vi "Dashboard Main.vi"() -> ()   [LabVIEW 2015]
uses:
  Camera Types.ctl
  <vilib>/Utility/miscctls.llb/LVRowAndColumnTypeDef.ctl
  <vilib>/event_ctls.llb/eventvkey.ctl
  <vilib>/Rock Robotics/WPI/Dashboard/WPI_DashboardLogging Global.vi
  <vilib>/Utility/file.llb/Write Delimited Spreadsheet (DBL).vi
  <vilib>/Rock Robotics/Network Tables/NT Write Numeric Array.vi
  <vilib>/Utility/file.llb/Read Delimited Spreadsheet (DBL).vi
  <vilib>/Rock Robotics/Network Tables/NT Read Boolean.vi
  <vilib>/Utility/config.llb/Write Key (String).vi
  <vilib>/Utility/config.llb/Write Key (I32).vi
  <vilib>/Utility/config.llb/NI_LVConfig.lvlib
  <vilib>/vision/NI_Vision_Development_Module.lvlib
panel:
  in  "Dashboard Tab":T1(tab)=enum."Camera Settings"
  out "Have ball?":bool
  out "Gyro":dbl
  in  "Camera Settings":T2={"Frame Rate"=30, "Compression"=30, "Size"=1} {"Frame Rate" scale=1.0..30.0; "Size" items=["640x480", "320x240", "160x120"]}
  out "Mode":T3(ring)=enum."Auto Disabled"
  in  "DB Camera Config":bool
  out "fps":dbl format="%#.1g"
  out "Mbps":dbl format="%#.1g"
  out "Mbps LED":bool
  in  "Auto Position":i32(slide)=1 scale=1.0..5.0
  in  "Auto Defense":T4(ring)=enum."Low Bar"
  out "TARGET":dbl
  in  "Test Slider":dbl(slide) scale=0.0..100.0 scale format="%#_3g"
  in  "On/Off":bool caption="Solenoid"
  in  "Test Name":u16(ring) items=["Select the test to run..."]
  in  "Test Tree":string(tree)
  in  "Motor":cluster{"Value":dbl, "Enable":bool} {"Value" scale=-1.0..1.0 scale format="%#_3g"}
  out "Progress":T5 {"Test Progress" scale=0.0..100.0}
  in  "Rev/Fwd":cluster{"Forward":bool, "Reverse":bool}
  in  "Test Ring":u16(ring) items=["Monochrome", "Color"]
  out "Cmd Status":string
  in  "Execute Command":bool
  in  "Command Params":string[][](table)
  in  "Command Selection":i32(listbox)
  out "NT Connection":bool
  in  "Select Auto":string(combo)
  in  "CheckList":i32(listbox)
  out "Detected Targets":T6(array[cluster]) {"Normalized Rect"."Numeric 5" format="%#_2g"; "Normalized Rect"."Numeric 3" format="%#_2g"; "Normalized Rect"."Numeric 2" format="%#_2g"; "Normalized Rect"."Numeric" format="%#_2g"}
  out "Masked":T7(plugin-control)
  out "Background":bool
  out "Qualified Particles":i32
  out "Highest Avg Score":dbl format="%#_3g"
  in  "Std Devs for Calibration":cluster{"H":dbl, "S":dbl, "V":dbl}={"H"=4.0, "S"=6.0, "V"=6.0}
  in  "Rec Mode":enum32{"Stop", "Record", "Playback"}(radio)
  in  "LED Color":T8={"Hue"={110.52399131877658, 148.6727294921875}, "Sat"={34.78571428571429, 255.0}, "Val"={91.07142857142858, 255.0}} {"Hue" scale=0.0..255.0 scale format="%_1f"}
  in  "Annotate":bool=TRUE
  in  "Annotation Limit":dbl=75.0
  in  "Aspect Ratio Fudge Factor":dbl=1.0
  in  "Min Score Threshold":i32=70
  in  "Camera Type":T9=enum."1013"
  in  "Emphasize Limit Tests":bool=TRUE
  in  "Green BCG Values":T10={"Brightness"=128.0, "Contrast"=45.0, "Gamma"=1.0} {"Brightness" min=0 max=255 step=1 format="%.2f"; "Contrast" min=1 max=89 step=1 format="%.2f"; "Gamma" min=0.1 max=10 step=0.01 format="%.2f"}
  in  "Blue BCG Values":T10={"Brightness"=128.0, "Contrast"=45.0, "Gamma"=1.0} {"Brightness" min=0 max=255 step=1 format="%.2f"; "Contrast" min=1 max=89 step=1 format="%.2f"; "Gamma" min=0.1 max=10 step=0.01 format="%.2f"}
  in  "Red BCG Values":T10={"Brightness"=128.0, "Contrast"=45.0, "Gamma"=1.0} {"Brightness" min=0 max=255 step=1 format="%.2f"; "Contrast" min=1 max=89 step=1 format="%.2f"; "Gamma" min=0.1 max=10 step=0.01 format="%.2f"}
  in  "Vision":u16(ring) items=["Camera Off", "USB Camera SW", "USB Camera HW", "IP Camera"]
  in  "Save?":bool
  out "Tree":string(tree)
  out "Original Image":T7(plugin-control)
  out "Camera Image":T7(plugin-control)
  in  "TCP":refnum<k5>
  out "Camera IP":string
  out "Image Message":string="Timeout in Camera Communications"
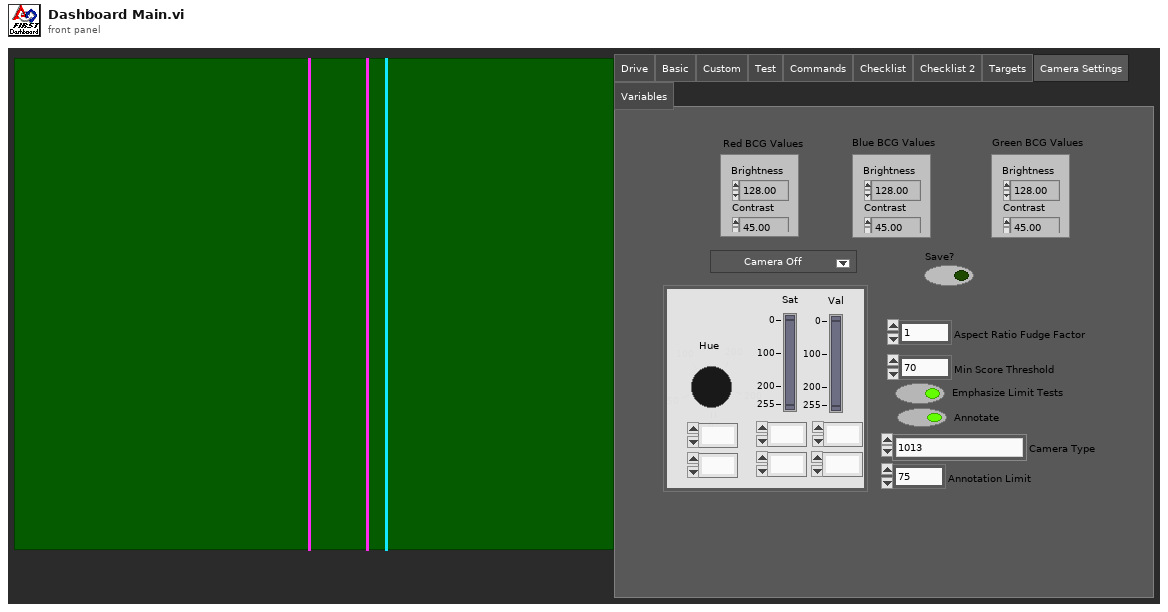
[diagram p1: front panel]
types:
  T1 = enum32{"Drive", "Basic", "Custom", "Test", "Commands", "Checklist", "Checklist 2", "Targets", "Camera Settings", "Variables"}
  T2 = cluster{"Frame Rate":i32, "Compression":i32, "Size":u16}
  T3 = enum8{"Tele-Op Disabled", "Tele-Op Enabled", "Auto Disabled", "Auto Enabled", "Test Disabled", "Test Enabled", "Disconnected", "No Code", "E-Stop"}
  T4 = enum16{"Portcullis", "Cheval de Frise", "Low Bar", "Rock Wall", "Rough Terrain", "Moat", "Ramparts", "2-ball"}
  T5 = cluster{"Test Progress":u8, "Test Progress Text":string}
  T6 = cluster{"Distance (ft)":dbl, "Center":cluster{dbl, dbl}, "Normalized Rect":cluster{"Numeric":dbl, "Numeric 2":dbl, "Numeric 3":dbl, "Numeric 5":dbl}}[]
  T7 = typedef "IMAQ Image.ctl" = refnum<image>
  T8 = cluster{"Hue":cluster{dbl, dbl}, "Sat":cluster{dbl, dbl}, "Val":cluster{dbl, dbl}}
  T9 = typedef "Camera Types.ctl" = enum16{"206", "1011", "1013", "MS HD3000 square", "MS HD3000 640x480"}
  T10 = cluster{"Brightness":sgl, "Contrast":sgl, "Gamma":sgl}
  T11 = typedef "Image Type" = u32
  T12 = cluster{"IDs":cluster{"RPC field ID":u16, "Unique ID":u16}, "String":string}
  T13 = enum32{"Drive", "Basic", "Custom", "Test", "Checklist", "Variables"}
  T14 = cluster{cluster{"Numeric":dbl, "Numeric":dbl}, cluster{"Numeric":dbl, "Numeric":dbl}, cluster{"Numeric":dbl, "Numeric":dbl}}
  T15 = cluster{"Camera Image":refnum<vi>, "Dashboard Tab":refnum<vi>, "Background":refnum<vi>, "Vision":refnum<vi>, "Rec Mode":refnum<vi>, "Test Slider":refnum<vi>, "On/Off ":refnum<vi>, "Test Ring":refnum<vi>, "Rev/Fwd":refnum<vi>, "Test Name":refnum<vi>, "Motor":refnum<vi>, "Progress":refnum<vi>, "CheckList":refnum<vi>, "Tree":refnum<vi>, "Test Tree":refnum<vi>, "Command Params":refnum<vi>, "Command Selection":refnum<vi>, "Execute Command":refnum<vi>, "Cmd Status":refnum<vi>}
  T16 = typedef "Particle Parameters" = i32
  T17 = cluster{cluster{dbl, dbl}, cluster{dbl, dbl}, cluster{dbl, dbl}}
  T18 = cluster{"Bounding box":cluster{"left":dbl, "top":dbl, "right":dbl, "bottom":dbl}, "Aspect Ratio":dbl, "Area to CH":dbl, "X Mask":dbl, "Y Mask":dbl, "Moment":dbl}[]
  T19 = cluster{"Distance (ft)":dbl, "Center":cluster{dbl, dbl}, "Normalized Rect":cluster{"Numeric":dbl, "Numeric 2":dbl, "Numeric 3":dbl, "Numeric 5":dbl}}
  T20 = cluster{"Numeric":dbl, "Numeric 2":dbl, "Numeric 3":dbl, "Numeric 5":dbl}
  T21 = typedef "NI_LVConfig.lvlib/Config Data RefNum.ctl" = refnum<k1>
  T22 = cluster{"Error Strings":string, "Disable Counts":cluster{u16, u16}, "Rail Faults":cluster{u16, u16, u16}, "Robot IP":string, "DB Mode":u8, "Event Info":cluster{"Name":string, "Type":u8, "Number":u16, "Replay":u8}, "Camera Addr":string}
  T23 = cluster{"Storage":cluster{"Disk Free":u64, "RAM Block":u32, "RAM free":u32}, "CPU Utilization":cluster{"CPU % ISR":sgl, "CPU % Time Crit":sgl, "CPU % Timed Str":sgl, "CPU % High":sgl, "CPU % Above":sgl, "CPU % Normal":sgl, "CPU % Low":sgl}, "CAN":cluster{"% Bus Utilization":sgl, "Bus Off Cnt":u32, "TX_FIFO Full Cnt":u32, "Receive Error Cnt":u8, "Transmit Error Cnt":u8}, "HID":cluster{"HID Outputs":u32, "Rumble Low":u16, "Rumble High":u16}[]}
  T24 = cluster{"Status bits":cluster{"Test Mode":bool, "Autonomous":bool, "Enabled":bool, "Code Start":bool, "Brownout":bool, "Reserved 2":bool, "Reserved 3":bool, "E-Stop":bool}, "Code Trace":cluster{"Disabled":bool, "TeleOp":bool, "Auto":bool, "Test":bool}, "Controller Type":enum16{"unknown", "cRIO", "roboRio"}, "Code?":enum16{"unknown", "noCode", "code"}, "Battery V":dbl}
  T25 = cluster{"Control Bits":cluster{"TestMode":bool, "Autonomous":bool, "Enabled":bool, "FMS Present":bool, bool, bool, bool, "E-Stop":bool}, "Team Station ":u8, "Countdown":sgl, "Joystick Values":cluster{"Axes":dbl[], "Buttons":bool[], "POVs":i16[]}[]}
  T26 = cluster{"Operation":enum16{"Update", "Clear"}, "Color Box":u32}[]
  T27 = typedef "eventvkey.ctl" = enum16{"ASCII", "Enter", "Return", "Shift", "Ctrl", "Alt", "Cmd", "Opt", "Caps", "NumLock", "Clear", "Break", "Up", "Down", "Left", "Right", "Insert", "Delete", "Home", "End", "PageUp", "PageDown", "Escape", "Help", "Pause", "ScrollLock", "F1", "F2", "F3", "F4", "F5", "F6", "F7", "F8", "F9", "F10", "F11", "F12", "F13", "F14", "F15", "F16", "F17", "F18", "F19", "F20", "F21", "F22", "F23", "F24", "Play", "VolumeUp", "VolumeDown", "Mute", "Two Byte Char"}
  T28 = cluster{"Image Size":bool, "Image Type":bool, "Pixel Value":bool, "ROI Information":bool, "Zoom Factor":bool}
  T29 = enum8{"Enabled", "Disabled", "Disabled and Grayed Out"}
  T30 = cluster{"Operation":enum16{"Update", "Clear"}, "Color Box":u32}
  T31 = typedef "LVRowAndColumnTypeDef.ctl" = cluster{"Row":i32, "Column":i32}
  T32 = cluster{"Shift":bool, "Ctrl":bool, "Alt":bool, "Cmd":bool, "Opt":bool}
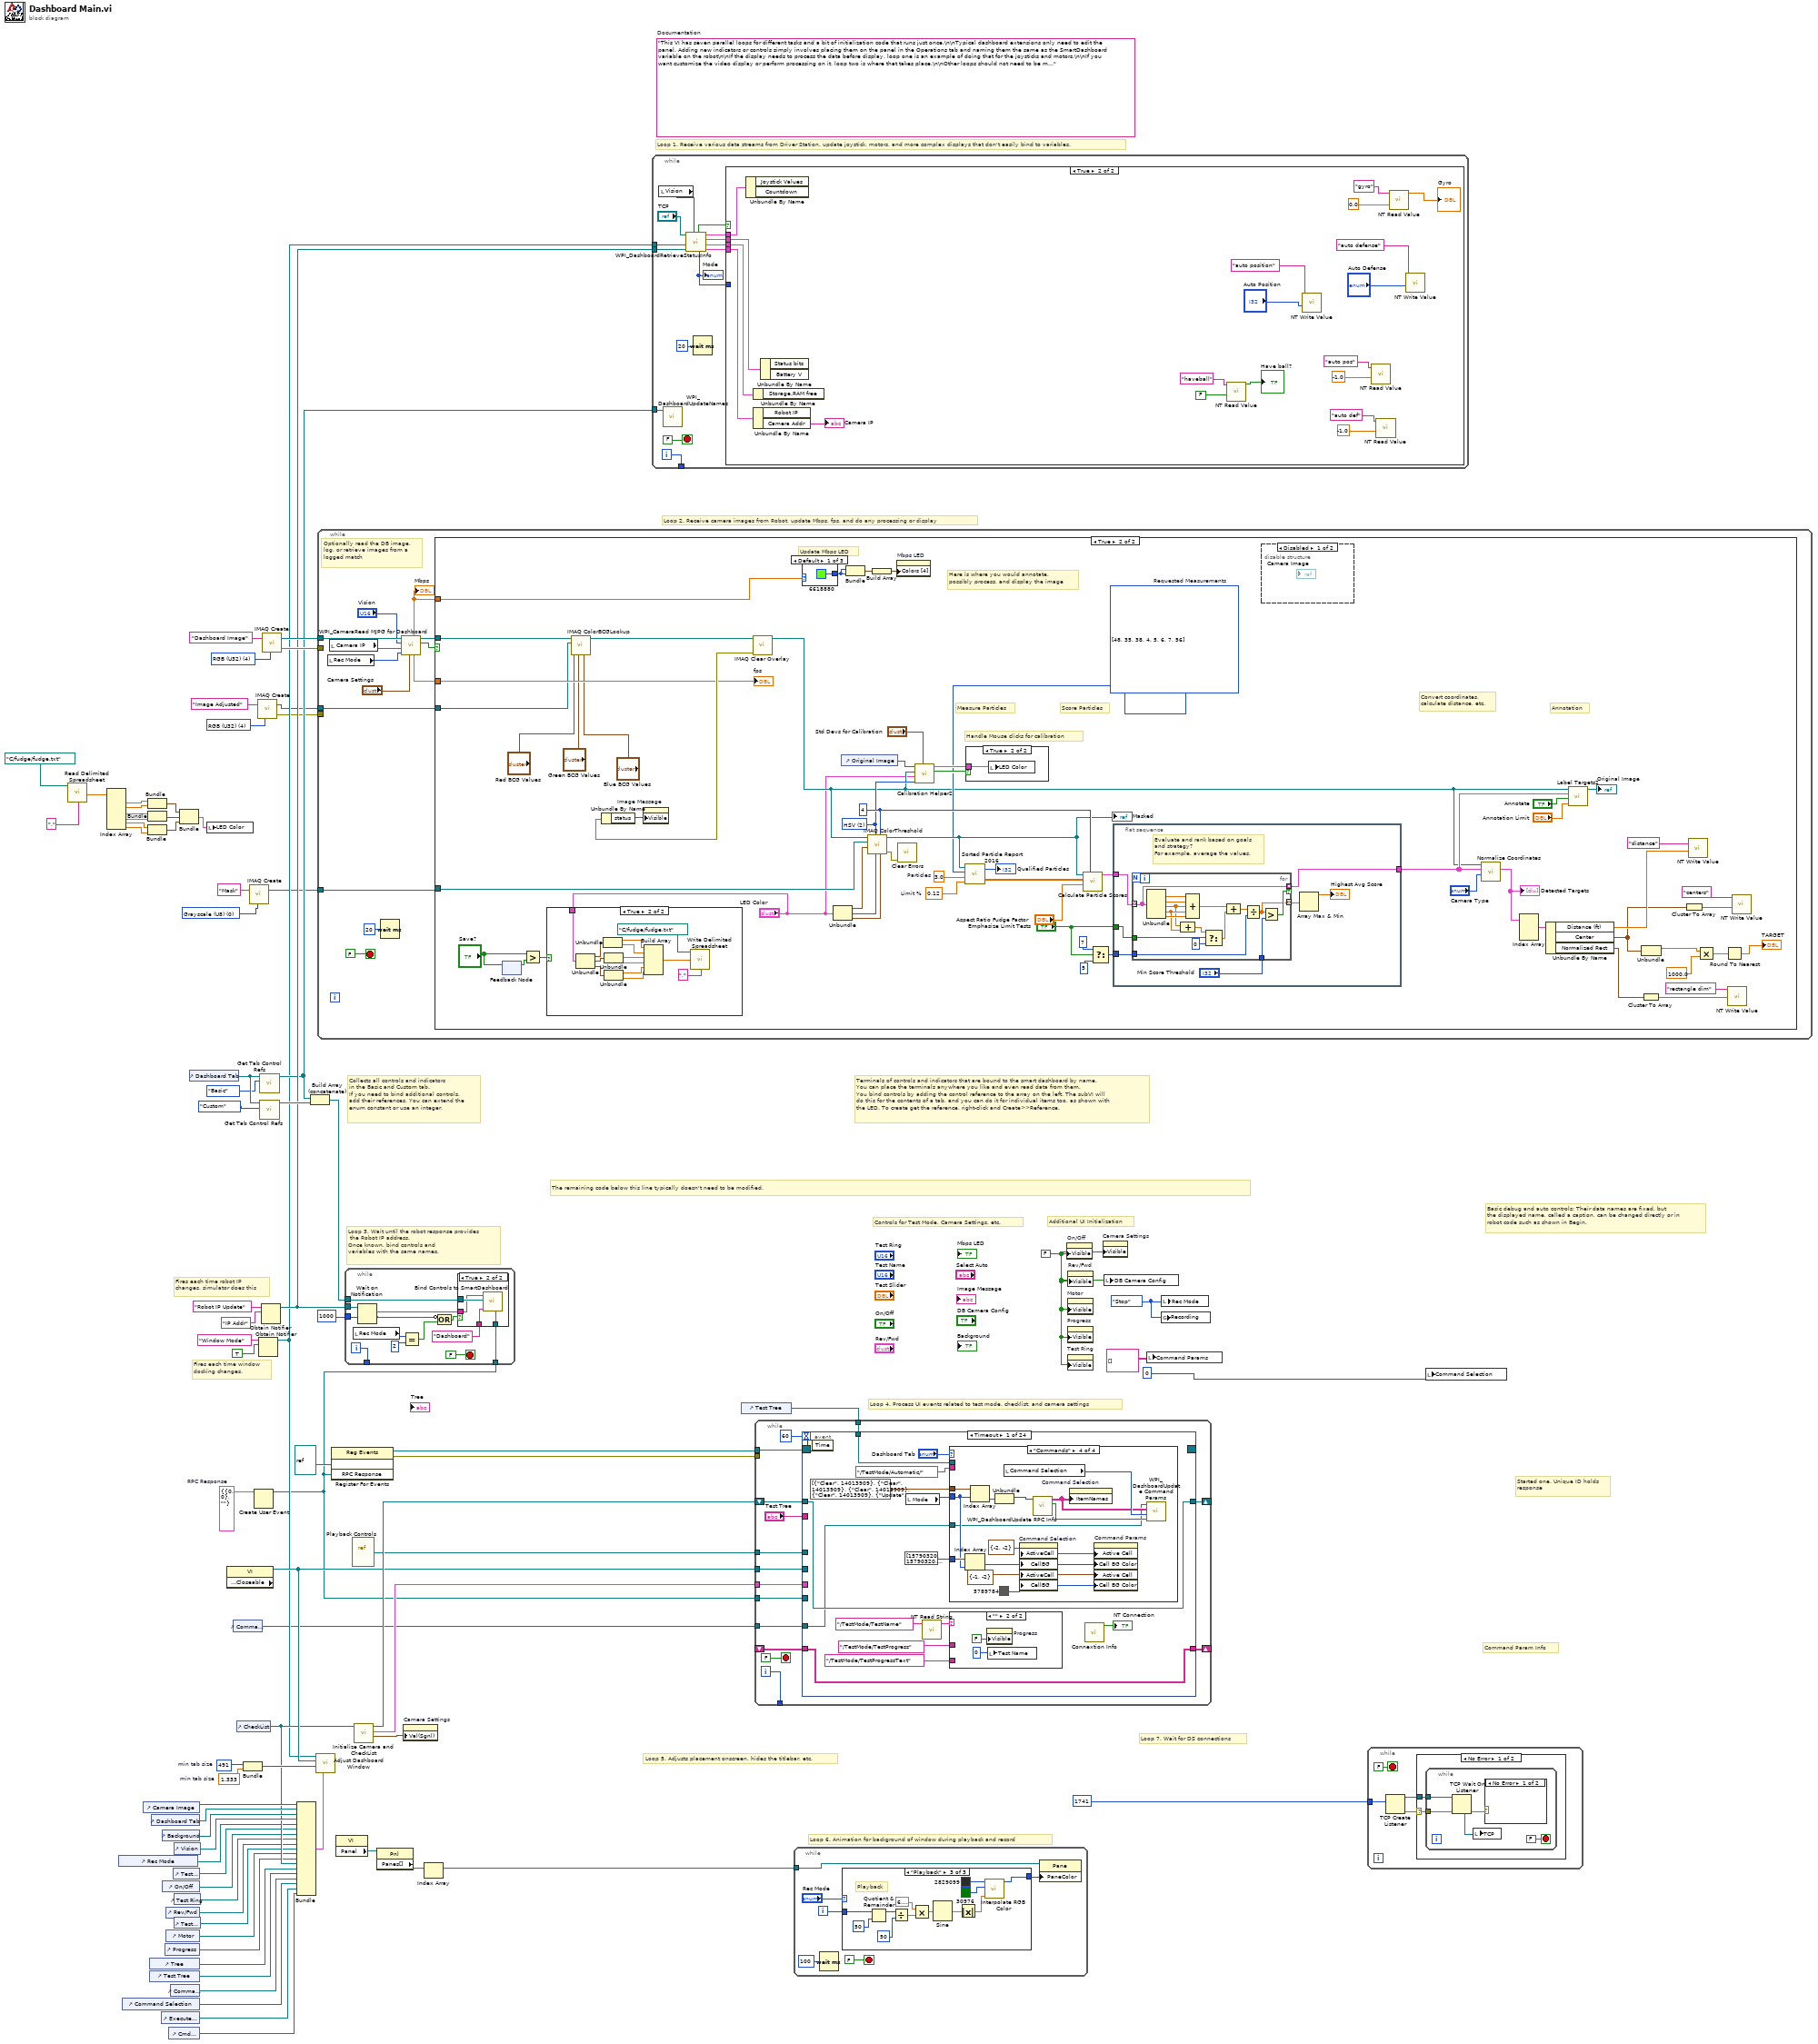
[diagram p0: block diagram]
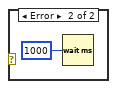
[diagram p2: hidden frame]
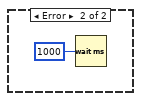
[diagram p3: hidden frame]
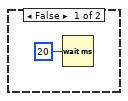
[diagram p4: hidden frame]
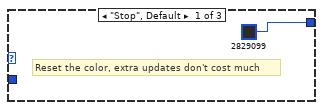
[diagram p5: hidden frame]
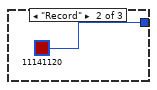
[diagram p6: hidden frame]
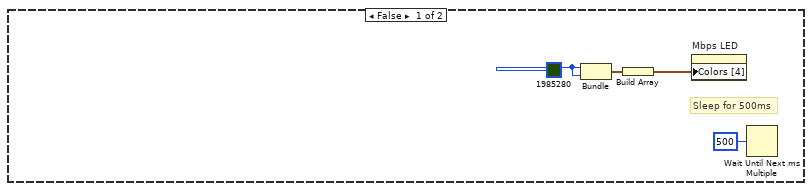
[diagram p8: hidden frame]
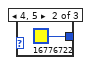
[diagram p12: hidden frame]
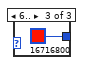
[diagram p13: hidden frame]
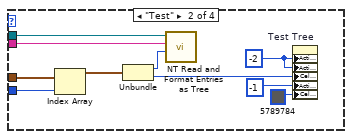
[diagram p15: hidden frame]
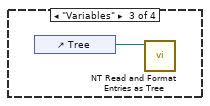
[diagram p16: hidden frame]
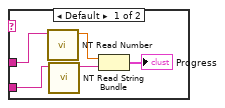
[diagram p17: hidden frame]
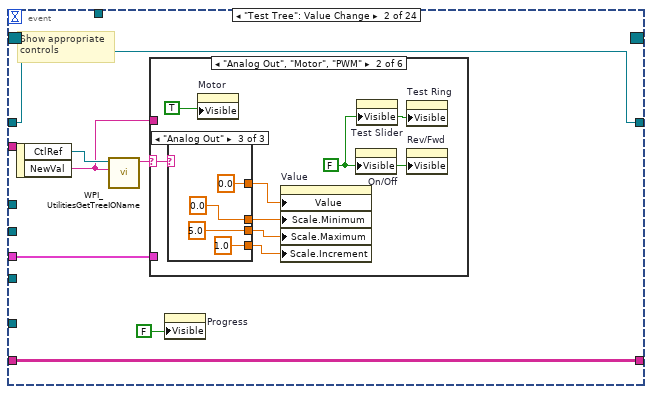
[diagram p18: hidden frame]
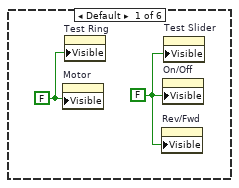
[diagram p19: hidden frame]
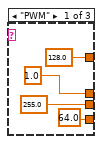
[diagram p20: hidden frame]
diagram:
  w17 = T11 4 items=["Grayscale (U8)", "Grayscale (I16)", "Grayscale (SGL)", "Complex (CSG)", "RGB (U32)", "HSL (U32)", "RGB (U64)"] ("Image Type")
  w19 = T11 0 items=["Grayscale (U8)", "Grayscale (I16)", "Grayscale (SGL)", "Complex (CSG)", "RGB (U32)", "HSL (U32)", "RGB (U64)", "Grayscale (U16)"] ("Image Type")
  w27 = T12 {"IDs"={"RPC field ID"=0, "Unique ID"=0}, "String"=""}  # RPC Response
  w52 = 491  # min tab size
  w51 = 1.333  # min tab size
  w60 = enum32{"Stop", "Record", "Playback"}."Stop" ("Rec Mode")
  w34 = FALSE ("Visible")
  (unwired) "This VI has seven parallel loops for different tasks and a bit of initialization code that runs just once.\n\nTypical dashboard extensions only need to edit the panel. Adding new indicators or controls simply involves placing them on the panel in the Operations tab and naming them the same as the SmartDashboard variable on the robot\n\nIf the display needs to process the data before display, loop one is an example of doing that for the joysticks and motors.\n\nIf you want customize the video display or perform processing on it, loop two is where that takes place.\n\nOther loops should not need to be modified. They are pretty standard, and document the task they perform."  # Documentation
  w80 = T11 4 items=["Grayscale (U8)", "Grayscale (I16)", "Grayscale (SGL)", "Complex (CSG)", "RGB (U32)", "HSL (U32)", "RGB (U64)"] ("Image Type")
  # "Command Param Info"
  # "Started one, Unique ID holds\nresponse"
  # "Loop 7. Wait for DS connections"
  # "Basic debug and auto controls: Their data names are fixed, but\nthe displayed name, called a caption, can be changed directly or in\nrobot code such as shown in Begin."
  # "Controls for Test Mode, Camera Settings, etc."
  # "Additional UI Initialization"
  # "Loop 6. Animation for background of window during playback and record"
  # "Fires each time robot IP\nchanges, simulator does this"
  # "Fires each time window\ndocking changes."
  # "Collects all controls and indicators\nin the Basic and Custom tab.\nIf you need to bind additional controls,\nadd their references. You can extend the\nenum constant or use an integer."
  # "The remaining code below this line typically doesn't need to be modified."
  # "Loop 4. Process UI events related to test mode, checklist, and camera settings"
  # "Terminals of controls and indicators that are bound to the smart dashboard by name.\nYou can place the terminals anywhere you like and even read data from them.\nYou bind controls by adding the control reference to the array on the left. The subVI will\ndo this for the contents of a tab, and you can do it for individual items too, as shown with\nthe LED. To create get the reference, right-click and Create>>Reference."
  # "Loop 3. Wait until the robot response provides\n the Robot IP address.\nOnce known, bind controls and\nvariables with the same names."
  # "Loop 5. Adjusts placement onscreen, hides the titlebar, etc."
  # "Loop 1. Receive various data streams from Driver Station, update joystick, motors, and more complex displays that don't easily bind to variables."
  # "Loop 2. Receive camera images from Robot, update Mbps, fps, and do any processing or display"
  n1 = call-poly <vilib>:"Read Delimited Spreadsheet.vi"("file path (dialog if empty)"=path "C:/fudge/fudge.txt", "delimiter (\\t)"="," ("delimiter (\\t)")) -> ("first row"=w11:dbl[])  [unwired: 8 in, 5 out]
  n2 = Index Array(array=w11) -> (element #1=w10:dbl, element #2=w9:dbl, element #3=w8:dbl, element #4=w7:dbl, element #5=w6:dbl, element #6=w5:dbl)  [unwired: 6 in]
  n3 = control-ref of="Rec Mode"() -> (w40:refnum<vi>)
  n4 = control-ref of="Command Selection"() -> (w26:refnum<vi>)
  n5 = control-ref of="Camera Image"() -> (w55:refnum<vi>)
  n6 = Bundle("Numeric"=w10, "Numeric"=w9) -> (w4:cluster{"Numeric":dbl, "Numeric":dbl})  [unwired: 1 in]
  n7 = Bundle("Numeric"=w8, "Numeric"=w7) -> (w3:cluster{"Numeric":dbl, "Numeric":dbl})  [unwired: 1 in]
  n8 = Bundle("Numeric"=w6, "Numeric"=w5) -> (w2:cluster{"Numeric":dbl, "Numeric":dbl})  [unwired: 1 in]
  n9 = control-ref of="Tree"() -> (w44:refnum<vi>)
  n10 = control-ref of="Test Tree"() -> (w43:refnum<vi>)
  n11 = control-ref of="Dashboard Tab"() -> (w54:refnum<vi>)
  n12 = control-ref of="Execute Command"() -> (w28:refnum<vi>)
  n13 = control-ref of="Background"() -> (w49:refnum<vi>)
  n14 = control-ref of="On/Off"() -> (w38:refnum<vi>)
  n15 = control-ref of="Progress"() -> (w35:refnum<vi>)
  n16 = control-ref of="Rev/Fwd"() -> (w36:refnum<vi>)
  n17 = control-ref of="Motor"() -> (w41:refnum<vi>)
  n18 = control-ref of="Cmd Status"() -> (w22:refnum<vi>)
  n19 = control-ref of="Command Params"() -> (w29:refnum<vi>)
  n20 = control-ref of="Test Slider"() -> (w39:refnum<vi>)
  n21 = control-ref of="Vision"() -> (w53:refnum<vi>)
  n22 = control-ref of="Test Ring"() -> (w37:refnum<vi>)
  n23 = control-ref of="Test Name"() -> (w42:refnum<vi>)
  n24 = Bundle(w4, w3, w2) -> (w1:T14)  [unwired: 1 in]
  n25 = control-ref of="Dashboard Tab"() -> (w58:refnum<vi>)
  n26 = local write "LED Color"(w1) -> ()
  n27 = property class="VI" props=["Front Panel.Closeable"]() -> (reference out=w59:refnum<vi>)  [unwired: 2 in, 2 out]
  n28 = control-ref of="Command Params"() -> (w21:refnum<vi>)
  n29 = control-ref of="CheckList"() -> (w45:refnum<vi>)
  n30 = Bundle("min tab size"=w52, "min tab size"=w51) -> (w50:cluster{"min tab size":i32, "min tab size":dbl})  [unwired: 1 in]
  n31 = call "IMAQ Create"("Image Name"="Mask", "Image Type"=w19) -> ("New Image"=w18:T7)  [unwired: 2 in, 2 out]
  n32 = Create User Event(user event datatype=w27) -> (user event=w23:refnum<user-event>)  [unwired: 1 in, 1 out]
  n33 = call "IMAQ Create"("Image Name"="Image Adjusted", "Image Type"=w17) -> ("New Image"=w15:T7, "error out"=w14:errorcluster)  [unwired: 2 in, 1 out]
  n34 = Obtain Notifier(name (unnamed)="Window Mode", notification data type=TRUE) -> (notifier out=w31:refnum<notifier>)  [unwired: 2 in, 2 out]
  n35 = call <vilib>:"Get Tab Control Refs.vi"("Page Index"=T13."Basic" ("Dashboard Tab"), "TabControl in"=w58) -> ("ControlsOnPage"=w32:refnum<vi>[])  [unwired: 9 in]
  n36 = call <vilib>:"Get Tab Control Refs.vi"("Page Index"=T13."Custom" ("Dashboard Tab"), "TabControl in"=w58) -> ("ControlsOnPage"=w57:refnum<vi>[])  [unwired: 9 in]
  n37 = Obtain Notifier(name (unnamed)="Robot IP Update", notification data type="IP Addr" ("name (unnamed)")) -> (notifier out=w33:refnum<notifier>)  [unwired: 2 in, 2 out]
  n38 = call "IMAQ Create"("Image Name"="Dashboard Image", "Image Type"=w80) -> ("New Image"=w78:T7, "error out"=w77:errorcluster)  [unwired: 2 in, 1 out]
  n39 = Bundle("Camera Image"=w55, "Dashboard Tab"=w54, "Background"=w49, "Vision"=w53, "Rec Mode"=w40, "Test Slider"=w39, "On/Off"=w38, "Test Ring"=w37, "Rev/Fwd"=w36, "Test Name"=w42, "Motor"=w41, "Progress"=w35, "CheckList"=w45, "Tree"=w44, "Test Tree"=w43, "Command Params"=w29, "Command Selection"=w26, "Execute Command"=w28, "Cmd Status"=w22) -> (w46:T15)  [unwired: 1 in]
  n40 = Build Array (concatenate)(w32, w57) -> (w56:refnum<vi>[])
  n41 = call "Adjust Dashboard Window.vi"("Sizing Refnums"=w46, "Size Constraints"=w50, "VI"=w59, "WIn Mode"=w31) -> ()  [unwired: 8 in]
  n42 = while {
    tunnel: w78 -> [w93]
    tunnel: w77 -> [_]
    tunnel: w18 -> [w83]
    tunnel: w15 -> [w82]
    tunnel: w14 -> [_]
    stop <- FALSE stop-if-true
    # "Optionally read the DB image,\nlog, or retrieve images from a\nlogged match"
    n43 = local read "Rec Mode"() -> (w88:enum32{"Stop", "Record", "Playback"})
    n44 = local read "Camera IP"() -> (w86:string)
    n45 = Wait (ms)(milliseconds to wait=u32 20) -> ()  [unwired: 1 out]
    n46 = call <vilib>:"WPI_CameraRead MJPG for Dashboard.vi"("Camera Settings"="Camera Settings", "Rec Mode"=w88, "Camera IP"=w86, "Camera Mode"="Vision", "Refnum in"=w93) -> ("Active"=w91:bool, "Refnum out"=w92:T7, "FPS"=w90:dbl, "Bandwidth (Mbps)"=w85:dbl)  [unwired: 3 in]
    "Mbps" <- w85
    n47 = case shown="True" w91 {
      tunnel: w92 -> [_ w121]
      tunnel: w85 -> [_ w152]
      tunnel: w90 -> [_ w151]
      tunnel: w83 -> [_ w125]
      tunnel: w82 -> [_ w119]
      frame False {
        w94 = u32 1985280 ("Color Box")
        # "Sleep for 500ms"
        n48 = Bundle("Color Box"=w94, "Color Box"=w94) -> (w96:cluster{"Color Box":u32, "Color Box":u32})  [unwired: 1 out]
        n49 = Build Array(w96) -> (w95:cluster{"Color Box":u32, "Color Box":u32}[])
        n50 = property on="Mbps LED" class="Bool (strict)"("Colors [4]"=w95) -> ()  [unwired: 2 in, 2 out]
        n51 = Wait Until Next ms Multiple(millisecond multiple=u32 500) -> ()  [unwired: 1 out]
      }
      frame True {
        w124 = T16[] [48, 35, 38, 4, 5, 6, 7, 56] items=["Center of Mass X", "Center of Mass Y", "First Pixel X", "First Pixel Y", "Bounding Rect Left", "Bounding Rect Top", "Bounding Rect Right", "Bounding Rect Bottom", "Max Feret Diameter Start X", "Max Feret Diameter Start Y", "Max Feret Diameter End X", "Max Feret Diameter End Y", "Max Horiz. Segment Length Left", "Max Horiz. Segment Length Right", "Max Horiz. Segment Length Row", "-", "Bounding Rect Width", "Bounding Rect Height", "Bounding Rect Diagonal", "Perimeter", "Convex Hull Perimeter", "Holes' Perimeter", "Max Feret Diameter", "Equivalent Ellipse Major Axis", "Equivalent Ellipse Minor Axis", "Equivalent Ellipse Minor Axis (Feret)", "Equivalent Rect Long Side", "Equivalent Rect Short Side", "Equivalent Rect Diagonal", "Equivalent Rect Short Side (Feret)", "Average Horiz. Segment Length", "Average Vert. Segment Length", "Hydraulic Radius", "Waddel Disk Diameter", "-", "Area", "Holes' Area", "Particle & Holes' Area", "Convex Hull Area", "Image Area", "-", "Number of Holes", "Number of Horiz. Segments", "Number of Vert. Segments", "-", "Orientation", "Max Feret Diameter Orientation", "-", "% Area/Image Area", "% Area/(Particle & Holes' Area)", "Ratio of Equivalent Ellipse Axes", "Ratio of Equivalent Rect Sides", "-", "Elongation Factor", "Compactness Factor", "Heywood Circularity Factor", "Type Factor", "-", "Sum X", "Sum Y", "Sum XX", "Sum XY", "Sum YY", "Sum XXX", "Sum XXY", "Sum XYY", "Sum YYY", "-", "Moment of Inertia XX", "Moment of Inertia XY", "Moment of Inertia YY", "Moment of Inertia XXX", "Moment of Inertia XXY", "Moment of Inertia XYY", "Moment of Inertia YYY", "Norm. Moment of Inertia XX", "Norm. Moment of Inertia XY", "Norm. Moment of Inertia YY", "Norm. Moment of Inertia XXX", "Norm. Moment of Inertia XXY", "Norm. Moment of Inertia XYY", "Norm. Moment of Inertia YYY", "Hu Moment 1", "Hu Moment 2", "Hu Moment 3", "Hu Moment 4", "Hu Moment 5", "Hu Moment 6", "Hu Moment 7"]  # Requested Measurements
        w142 = 4 ("Replace Value")
        w144 = 0.12  # Limit %
        w147 = 3.0  # Particles
        w128 = u16 2 items=["RGB", "HSL", "HSV", "HSI"] ("Color Mode")
        # "Handle Mouse clicks for calibration"
        # "Measure Particles"
        # "Convert coordinates,\ncalculate distance, etc."
        # "Annotation"
        # "Score Particles"
        # "Here is where you would annotate,\npossibly process, and display the image"
        # "Update Mbps LED"
        n52 = feedback-in #1("Save?") -> ()
        n53 = feedback #1() -> (w100:bool)  [unwired: 1 in]
        n54 = Greater?(x="Save?", y=w100) -> (0:w101:bool)
        n55 = case shown="True" w101 {
          tunnel: "LED Color" -> [_ w162]
          frame False {
          }
          frame True {
            n56 = Unbundle(w162) -> ("Hue"=w164:cluster{dbl, dbl}, "Sat"=w163:cluster{dbl, dbl}, "Val"=w161:cluster{dbl, dbl})
            n57 = Unbundle(w164) -> (w170:dbl, w169:dbl)
            n58 = Unbundle(w163) -> (w168:dbl, w167:dbl)
            n59 = Unbundle(w161) -> (w166:dbl, w165:dbl)
            n60 = Build Array(w170, w169, w168, w167, w166, w165) -> (w159:dbl[])
            n61 = call-poly <vilib>:"Write Delimited Spreadsheet.vi"("file path (dialog if empty)"=path "C:/fudge/fudge.txt", "1D data"=w159, "delimiter (\\t)"="," ("delimiter (\\t)")) -> ()  [unwired: 11 in, 2 out]
          }
        }
        n62 = call "IMAQ ColorBCGLookup"("Blue BCG Values"="Blue BCG Values", "Green BCG Values"="Green BCG Values", "Red BCG Values"="Red BCG Values", "Image Dst"=w119, "Image Src"=w121) -> ("Image Dst Out"=w120:T7)  [unwired: 5 in, 1 out]
        n63 = call "IMAQ Clear Overlay"("Image"=w120) -> ("error out"=w156:errorcluster, "Image Out"=w122:T7)  [unwired: 2 in, 7 out]
        n64 = Unbundle By Name(w156) -> ("status"=w157:bool)
        n65 = property on="Image Message" class="Str"("Visible"=w157) -> ()  [unwired: 2 in, 2 out]
        n66 = case shown="Default" w152 {
          tunnel: [u32 6618880 ("Color Box") u32 16776722 ("Color Box") u32 16716800 ("Color Box")] -> w153
          frame Default {
          }
          frame 4, 5 {
          }
          frame 6.. {
          }
        }
        n67 = Unbundle("LED Color") -> ("Hue"=w150:cluster{dbl, dbl}, "Sat"=w149:cluster{dbl, dbl}, "Val"=w148:cluster{dbl, dbl})
        n68 = control-ref of="Original Image"() -> (w131:refnum<vi>)
        n69 = Bundle("Color Box"=w153, "Color Box"=w153) -> (w155:cluster{"Color Box":u32, "Color Box":u32})  [unwired: 1 out]
        n70 = call "IMAQ ColorThreshold"("Blue or Luma or Val or Inten Range"=w148, "Replace Value"=w142, "Green or Sat Range"=w149, "Color Mode"=w128, "Red or Hue Range"=w150, "Image Dst"=w125, "Image Src"=w122) -> ("error out"=w135:errorcluster, "Image Dst Out"=w136:T7)  [unwired: 3 in]
        "Masked" <- w136
        n71 = Build Array(w155) -> (w154:cluster{"Color Box":u32, "Color Box":u32}[])
        n72 = property on="Mbps LED" class="Bool (strict)"("Colors [4]"=w154) -> ()  [unwired: 2 in, 2 out]
        n73 = call <vilib>:"Clear Errors.vi"("error in (no error)"=w135) -> ()  [unwired: 5 in, 2 out]
        n74 = call "Calibration Helper2.vi"("Std Devs"="Std Devs for Calibration", "Color Mode"=w128, "Color Components"="LED Color", "Image"=w122, "Image Ctl Refnum"=w131) -> ("Changed"=w130:bool, "output color"=w129:T17)  [unwired: 5 in]
        n75 = call "Sorted Particle Report 2016.vi"("Min Area Size %"=w144, "Particle Count Limit"=w147, "Pixel Measurements"=w124, "Image in"=w136) -> ("Sorted Data"=w145:dbl[][], "Particles"=→"Qualified Particles":i32)
        n76 = case shown="True" w130 {
          tunnel: w129 -> [_ w171]
          frame False {
          }
          frame True {
            n77 = local write "LED Color"(w171) -> ()
          }
        }
        n78 = call "Calculate Particle Scores.vi"("Pixel Value"=w142, "Aspect Fudge Factor"="Aspect Ratio Fudge Factor", "Sorted Data"=w145, "Image in"=w136) -> ("Scores"=w139:T18)  [unwired: 7 in]
        n79 = Select(t=7, s="Emphasize Limit Tests", f=5) -> (s? t:f=w132:i32)
        n80 = flat-sequence {
          tunnel: w139 -> [w177]
          tunnel: [w178] -> w137
          tunnel: w132 -> [w174]
          tunnel: "Emphasize Limit Tests" -> [w172]
          frame #0 {
            # "Evaluate and rank based on goals\nand strategy?\nFor example, average the values."
            n81 = for {
              tunnel: w177 -> [w192] mode=indexing
              tunnel: [w192] -> w178 mode=indexing if=w191
              tunnel: [w190] -> w176 mode=indexing
              tunnel: w174 -> [w189]
              tunnel: "Min Score Threshold" -> [w188]
              tunnel: w172 -> [w181]
              n82 = Unbundle(w192) -> ("Aspect Ratio"=w194:dbl, "Area to CH"=w193:dbl, "X Mask"=w183:dbl, "Y Mask"=w184:dbl, "Moment"=w185:dbl)  [unwired: 1 out]
              n83 = Compound Arithmetic op=ADD(w183, w184) -> (w182:dbl)
              n84 = Compound Arithmetic op=ADD(w194, w193, w183, w184, w185) -> (w187:dbl)
              n85 = Select(t=w182, s=w181, f=0) -> (s? t:f=w180:dbl)
              n86 = Compound Arithmetic op=ADD(w187, w180) -> (w186:dbl)
              n87 = Divide(x=w186, y=w189) -> (x/y=w190:dbl)
              n88 = Greater?(x=w190, y=w188) -> (0:w191:bool)
            }
            n89 = Array Max & Min(array=w176) -> (max value=→"Highest Avg Score":dbl)  [unwired: 3 out]
          }
        }
        n90 = disable-structure shown="Disabled" {
          frame Disabled {
          }
          frame Enabled {
          }
        }
        n91 = call "Normalize Coordinates.vi"("Camera Type"="Camera Type", "Targets"=w137, "Image in"=w122) -> ("Found Targets"=w115:T6)  [unwired: 7 in, 1 out]
        "Detected Targets" <- w115
        n92 = Index Array(array=w115) -> (element #1=w114:T19)  [unwired: 3 in, 2 out]
        n93 = Unbundle By Name(w114) -> ("Distance (ft)"=w112:dbl, "Center"=w106:cluster{dbl, dbl}, "Normalized Rect"=w108:T20)
        n94 = call "Label Targets2.vi"("Score Threshold"="Annotation Limit", "Annotate"="Annotate", "Targets"=w137, "Image in"=w122) -> ("Image out"=→"Original Image":T7)  [unwired: 7 in]
        n95 = Cluster To Array(cluster=w108) -> (array=w107:dbl[])
        n96 = Unbundle(w106) -> (w102:dbl)  [unwired: 1 out]
        n97 = Cluster To Array(cluster=w106) -> (array=w110:dbl[])
        n98 = call-poly <vilib>:"NT Write Value.vi"("Numeric"=w112, "Name"="distance") -> ()  [unwired: 9 in, 1 out]
        n99 = Multiply(x=w102, y=1000.0) -> (x*y=w104:dbl)
        n100 = Round To Nearest(number=w104) -> (nearest integer value=→"TARGET":dbl)
        n101 = call-poly <vilib>:"NT Write Value.vi"("Numeric Array"=w107, "Name"="rectangle dim") -> ()  [unwired: 9 in, 1 out]
        n102 = call-poly <vilib>:"NT Write Value.vi"("Numeric Array"=w110, "Name"="centers") -> ()  [unwired: 9 in, 1 out]
        "fps" <- w151
      }
    }
  }
  n103 = register-events(refnum<vi> refnum, w23) -> (reference out=w64:refnum<event-registration>, error out=w63:errorcluster)  [unwired: 2 in]
  n104 = property class="VI"() -> ("Panel"=w67:refnum<vi>)  [unwired: 2 in, 2 out]
  n105 = while {
    tunnel: w56 -> [w210]
    tunnel: w33 -> [w208]
    tunnel: [w206] -> _
    tunnel: u32 1000 ("milliseconds to wait") -> [w205]
    tunnel: w23 -> [w198]
    i -> [w206]
    stop <- FALSE stop-if-true
    n106 = local read "Rec Mode"() -> (w201:enum32{"Stop", "Record", "Playback"})
    n107 = Wait on Notification(notifier=w208, timeout in ms (-1)=w205) -> (notification=w207:string, timed out?=w203:bool)  [unwired: 2 in, 2 out]
    n108 = Equal?(x=w201, y=u16 2 ("Rec Mode")) -> (x = y?=w202:bool)
    n109 = Compound Arithmetic op=OR(invert w203, w202) -> (w204:bool)
    n110 = case shown="True" w204 {
      tunnel: w210 -> [_ w214]
      tunnel: w207 -> [_ w213]
      tunnel: "Dashboard" -> [_ w212]
      tunnel: w198 -> [_ w211]
      frame False {
      }
      frame True {
        n111 = call <vilib>:"Bind Controls to SmartDashboard.vi"("RPC ref"=w211, "Client Name"=w212, "Bound Control Refs"=w214, "Server IP Address"=w213) -> ()  [unwired: 8 in]
      }
    }
  }
  n112 = vi-ref "Playback Controls.vi"() -> (w65:refnum<vi>)
  n113 = call "Initialize Camera and CheckList.vi"("ListBox in"=w45) -> ("Cluster"=w71:cluster{"value":i32, "value":i32, "index":i32}, "Array"=w72:cluster{string[]}[], "File Refnum"=w70:T21)  [unwired: 8 in]
  n114 = property class="Pnl"(reference=w67) -> ("Panes[]"=w68:refnum<vi>[])  [unwired: 1 in, 2 out]
  n115 = property on="Camera Settings" class="Clust (strict)"("Val(Sgnl)"=w71) -> ()  [unwired: 2 in, 2 out]
  n116 = Index Array(array=w68) -> (element=w66:refnum<vi>)  [unwired: 1 in]
  n117 = while {
    tunnel: [w227] -> _
    tunnel: w33 -> [w221]
    tunnel: w32 -> [w220]
    tunnel: w31 -> [w216]
    i -> [w227]
    stop <- FALSE stop-if-true
    n118 = local read "Vision"() -> (w218:u16)
    n119 = call <vilib>:"WPI_DashboardUpdateNames.vi"("Controls on Tab"=w220) -> ()  [unwired: 11 in]
    n120 = call <vilib>:"WPI_DashboardRetrieveStatusInfo.vi"("Vision"=w218, "Binding Refnum"=w221, "Window Mode Notifier"=w216, "TCP Cnx"="TCP") -> ("Power and Errors"=w222:T22, "Robot Metrics"=w225:T23, "Status Info"=w226:T24, "Control Info"=w223:T25, "Robot Mode"=w219:T3, "Process?"=w224:bool)  [unwired: 2 in]
    "Mode" <- w219
    n121 = Wait (ms)(milliseconds to wait=u32 20) -> ()  [unwired: 1 out]
    n122 = case shown="True" w224 {
      tunnel: w226 -> [_ w248]
      tunnel: w225 -> [_ w247]
      tunnel: w223 -> [_ w246]
      tunnel: w222 -> [_ w245]
      tunnel: w219 -> [_ _]
      frame False {
        n123 = Wait (ms)(milliseconds to wait=u32 20) -> ()  [unwired: 1 out]
      }
      frame True {
        n124 = Unbundle By Name(w246) -> ()  [unwired: 2 out]
        n125 = Unbundle By Name(w247) -> ()  [unwired: 1 out]
        n126 = Unbundle By Name(w245) -> ("Camera Addr"=→"Camera IP":string)  [unwired: 1 out]
        n127 = Unbundle By Name(w248) -> ()  [unwired: 2 out]
        n128 = call-poly <vilib>:"NT Read Value.vi"("Default Value"=FALSE, "Name"="haveball") -> ("Boolean"=→"Have ball?":bool)  [unwired: 8 in, 1 out]
        n129 = call-poly <vilib>:"NT Write Value.vi"("Numeric"="Auto Position", "Name"="auto position") -> ()  [unwired: 9 in, 1 out]
        n130 = call-poly <vilib>:"NT Read Value.vi"("Default Value"=-1.0, "Name"="auto pos") -> ()  [unwired: 8 in, 2 out]
        n131 = call-poly <vilib>:"NT Read Value.vi"("Default Value"=-1.0, "Name"="auto def") -> ()  [unwired: 8 in, 2 out]
        n132 = call-poly <vilib>:"NT Read Value.vi"("Default Value"=0.0, "Name"="gyro") -> ("Numeric"=→"Gyro":dbl)  [unwired: 8 in, 1 out]
        n133 = call-poly <vilib>:"NT Write Value.vi"("Numeric"="Auto Defense", "Name"="auto defense") -> ()  [unwired: 9 in, 1 out]
      }
    }
  }
  n134 = control-ref of="Test Tree"() -> (w69:refnum<vi>)
  n135 = while {
    tunnel: w72 -> [w260]
    shift-right: [w259] -> _
    shift-left: w70 -> [w258]
    tunnel: [w257] -> _
    tunnel: w69 -> [w256]
    tunnel: w65 -> [w255]
    tunnel: w64 -> [w254]
    tunnel: w63 -> [_]
    tunnel: w59 -> [w253]
    tunnel: w23 -> [w252]
    tunnel: w21 -> [w251]
    shift-right: [w250] -> _
    shift-left: _ -> [w249]
    i -> [w257]
    stop <- FALSE stop-if-true
    n136 = event shown="[0] Timeout" {
      selector: w254 -> [_ _ _ _ _ _ _ _ _ _ _ _ _ _ _ _ _ _ _ _ _ _ _ _]
      dyn-events: [_ _ _ _ _ _ _ _ _ _ _ _ _ _ _ _ _ _ w569 _ _ _ _ _] -> _
      timeout: u32 60 ("milliseconds to wait") -> [_ _ _ _ _ _ _ _ _ _ _ _ _ _ _ _ _ _ _ _ _ _ _ _]
      tunnel: w256 -> [w273 _ _ _ _ _ _ _ _ _ _ _ _ _ _ _ _ _ _ _ _ _ _ _]
      tunnel: "Test Tree" -> [_ _ _ _ _ _ _ _ _ _ _ _ _ w532 w541 w544 w549 w558 _ _ _ _ _ _]
      tunnel: w260 -> [_ w311 _ _ _ _ _ _ _ _ _ w494 w525 _ _ _ _ _ _ _ _ _ _ _]
      tunnel: [w270 w310 w414 w420 w430 w434 w440 w452 w460 w466 w479 w493 w518 w531 w539 w543 w548 w557 w571 w587 w589 w597 w608 w613] -> w259
      tunnel: w258 -> [w270 w310 w414 w420 w430 w434 w440 w452 w460 w466 w479 w492 w518 w531 w539 w543 w548 w557 w571 w587 w589 w597 w608 w613]
      tunnel: w255 -> [_ _ _ _ _ _ _ _ _ _ _ _ _ _ _ _ _ _ w572 _ w592 _ _ _]
      tunnel: w253 -> [_ _ _ _ _ _ _ _ _ _ _ _ _ _ _ _ _ _ w567 _ _ _ _ _]
      tunnel: w252 -> [_ _ _ _ _ _ _ _ _ _ _ _ _ _ _ _ _ _ w563 _ _ _ _ _]
      tunnel: w251 -> [w265 _ _ _ _ _ w438 _ _ _ _ _ _ _ _ _ _ _ _ _ _ _ _ _]
      tunnel: [w264 w309 w413 w419 w429 w435 w436 w446 w457 w465 w478 w491 w517 w530 w538 w542 w547 w556 w562 w585 w588 w593 w601 w614] -> w250
      tunnel: w249 -> [w264 w309 w413 w419 w429 w435 w436 _ _ w465 w478 w491 w517 w530 w538 w542 w547 w556 w562 w585 w588 w593 w601 w614]
      event Timeout {
        n137 = event-data() -> ()  [unwired: 1 in, 1 out]
        n138 = local read "Mode"() -> (w267:T3)
        n139 = call <vilib>:"NT Read String.vi"("Name"="/TestMode/TestName") -> ("String"=w276:string)  [unwired: 9 in, 1 out]
        n140 = case shown="\"Commands\"" "Dashboard Tab" {
          tunnel: w273 -> [_ w287 _ _]
          tunnel: "/TestMode/Automatic/" ("Name Pattern") -> [_ w286 _ _]
          tunnel: T26 [{"Operation"=enum."Clear", "Color Box"=14013909}, {"Operation"=enum."Clear", "Color Box"=14013909}, {"Operation"=enum."Clear", "Color Box"=14013909}, {"Operation"=enum."Clear", "Color Box"=14013909}, {"Operation"=enum."Update", "Color Box"=14013909}, {"Operation"=enum."Update", "Color Box"=16777215}, {"Operation"=enum."Clear", "Color Box"=14013909}, {"Operation"=enum."Clear", "Color Box"=14013909}, {"Operation"=enum."Clear", "Color Box"=14013909}] -> [_ w279 _ w296]
          tunnel: w267 -> [_ w278 _ w295]
          tunnel: u32[] [15790320, 15790320, 15790320, 15790320, 16777215, 16777215, 15790320, 15790320, 15790320] -> [_ _ _ w301]
          tunnel: w265 -> [_ _ _ w289]
          frame "Custom", Default {
          }
          frame "Test" {
            w285 = -2 ("Active Item:Row Number")
            n141 = Index Array(array=w279, index=w278) -> (element=w280:T30)
            n142 = Unbundle(w280) -> ("Operation"=w281:enum16{"Update", "Clear"}, "Color Box"=w282:u32)
            n143 = call <vilib>:"NT Read and Format Entries as Tree.vi"("Operation"=w281, "Name Pattern"=w286, "Tree Refnum"=w287) -> ()  [unwired: 7 in, 2 out]
            n144 = property on="Test Tree" class="Tree (strict)"("Active Item Row Number"=w285, "ActiveColNum"=w285, "CellBG"=w282, "Active Item Row Number"=-1 ("Active Item:Row Number"), "CellBG"=u32 5789784 ("Color Box")) -> ()  [unwired: 2 in, 2 out]
          }
          frame "Variables" {
            n145 = control-ref of="Tree"() -> (w288:refnum<vi>)
            n146 = call <vilib>:"NT Read and Format Entries as Tree.vi"("Tree Refnum"=w288) -> ()  [unwired: 9 in, 2 out]
          }
          frame "Commands" {
            w297 = u32 5789784 ("Color Box")
            w298 = T31 {"Row"=-1, "Column"=-2} ("Active Cell:Active Cell")
            w300 = T31 {"Row"=-2, "Column"=-2} ("Active Cell:Active Cell")
            n147 = Index Array(array=w301, index=w295) -> (element=w299:u32)
            n148 = Index Array(array=w296, index=w295) -> (element=w294:T30)
            n149 = Unbundle(w294) -> ("Operation"=w293:enum16{"Update", "Clear"})  [unwired: 1 out]
            n150 = local read "Command Selection"() -> (w292:i32)
            n151 = property on="Command Selection" class="MCListbox (strict)"("ActiveCell"=w300, "CellBG"=w299, "ActiveCell"=w298, "CellBG"=w297) -> ()  [unwired: 2 in, 2 out]
            n152 = call <vilib>:"WPI_DashboardUpdate RPC Info.vi"("Operation"=w293) -> ("update"=w291:bool, "commands"=w290:string[][])  [unwired: 9 in]
            n153 = property on="Command Selection" class="MCListbox (strict)"("ItemNames"=w290) -> ()  [unwired: 2 in, 2 out]
            n154 = property on="Command Params" class="Tbl (strict)"("Active Cell"=w300, "Cell BG Color"=w299, "Active Cell"=w298, "Cell BG Color"=w297) -> ()  [unwired: 2 in, 2 out]
            n155 = call <vilib>:"WPI_DashboardUpdate Command Params.vi"("Update"=w291, "NewVal"=w292, "Commands"=w290, "Param Tbl"=w289) -> ()  [unwired: 7 in, 1 out]
          }
        }
        n156 = case shown="\"\"" w276 {
          tunnel: "/TestMode/TestProgress" ("Name") -> [w303 _]
          tunnel: "/TestMode/TestProgressText" ("Name") -> [w302 _]
          frame Default {
            n157 = call <vilib>:"NT Read Number.vi"("Name"=w303) -> ("Numeric"=w304:dbl)  [unwired: 9 in, 1 out]
            n158 = call <vilib>:"NT Read String.vi"("Name"=w302) -> ("String"=w305:string)  [unwired: 9 in, 1 out]
            n159 = Bundle("Numeric"=w304, "String"=w305) -> (→"Progress":cluster{"Numeric":dbl, "String":string})  [unwired: 1 in]
          }
          frame "" {
            n160 = property on="Progress" class="Clust (strict)"("Visible"=FALSE) -> ()  [unwired: 2 in, 2 out]
            n161 = local write "Test Name"(u16 0) -> ()
          }
        }
        n162 = call <vilib>:"Connextion Info.vi"() -> ("Connected"=→"NT Connection":bool)  [unwired: 10 in, 1 out]
      }
      event "Test Tree": Value Change {
        # "Show appropriate\ncontrols"
        n163 = event-data() -> ("CtlRef"=w314:refnum<vi>, "NewVal"=w312:string)  [unwired: 1 in]
        n164 = call <vilib>:"WPI_UtilitiesGetTreeIOName.vi"("NewVal"=w312, "TreeControl in"=w314) -> ("I/O Name"=w315:string)  [unwired: 9 in]
        n165 = case shown="\"Analog Out\", \"Motor\", \"PWM\"" w315 {
          selector: w315 -> [_ w322 _ w344 w353 _]
          tunnel: w312 -> [_ _ w341 w343 _ w360]
          tunnel: w311 -> [_ _ _ _ _ w359]
          frame Default {
            w317 = FALSE ("Visible")
            w316 = FALSE ("Visible")
            n166 = property on="Motor" class="Clust (strict)"("Visible"=w316) -> ()  [unwired: 2 in, 2 out]
            n167 = property on="Test Ring" class="Ring (strict)"("Visible"=w316) -> ()  [unwired: 2 in, 2 out]
            n168 = property on="Rev/Fwd" class="Clust (strict)"("Visible"=w317) -> ()  [unwired: 2 in, 2 out]
            n169 = property on="On/Off" class="Bool (strict)"("Visible"=w317) -> ()  [unwired: 2 in, 2 out]
            n170 = property on="Test Slider" class="Slide (strict)"("Visible"=w317) -> ()  [unwired: 2 in, 2 out]
          }
          frame "Analog Out", "Motor", "PWM" {
            w323 = FALSE ("Visible")
            n171 = case shown="\"Analog Out\"" w322 {
              tunnel: [1.0 ("Value") -1.0 ("Value") 0.0 ("Value")] -> w321
              tunnel: [255.0 ("Value") 1.0 ("Value") 5.0 ("Value")] -> w320
              tunnel: [128.0 ("Value") 0.0 ("Value") 0.0 ("Value")] -> w319
              tunnel: [64.0 ("Value") 0.5 ("Value") 1.0 ("Value")] -> w318
              frame "PWM" {
              }
              frame "Motor", Default {
              }
              frame "Analog Out" {
              }
            }
            n172 = property on="Motor" class="Clust (strict)"("Visible"=TRUE) -> ()  [unwired: 2 in, 2 out]
            n173 = property on="Value" class="Slide (strict)"("Value"=w319, "Scale.Minimum"=w321, "Scale.Maximum"=w320, "Scale.Increment"=w318) -> ()  [unwired: 2 in, 2 out]
            n174 = property on="On/Off" class="Bool (strict)"("Visible"=w323) -> ()  [unwired: 2 in, 2 out]
            n175 = property on="Test Slider" class="Slide (strict)"("Visible"=w323) -> ()  [unwired: 2 in, 2 out]
            n176 = property on="Test Ring" class="Ring (strict)"("Visible"=w323) -> ()  [unwired: 2 in, 2 out]
            n177 = property on="Rev/Fwd" class="Clust (strict)"("Visible"=w323) -> ()  [unwired: 2 in, 2 out]
          }
          frame "Servo" {
            w339 = FALSE ("Visible")
            n178 = call <vilib>:"NT Read Number.vi"("Name"=w341) -> ("Numeric"=w340:dbl)  [unwired: 9 in, 1 out]
            n179 = property on="Test Slider" class="Slide (strict)"("Visible"=TRUE, "Scale.Maximum"=170.0 ("Scale.Range:Maximum")) -> ()  [unwired: 2 in, 2 out]
            n180 = local write "Test Slider"(w340) -> ()
            n181 = property on="Motor" class="Clust (strict)"("Visible"=w339) -> ()  [unwired: 2 in, 2 out]
            n182 = property on="Rev/Fwd" class="Clust (strict)"("Visible"=w339) -> ()  [unwired: 2 in, 2 out]
            n183 = property on="On/Off" class="Bool (strict)"("Visible"=w339) -> ()  [unwired: 2 in, 2 out]
            n184 = property on="Test Ring" class="Ring (strict)"("Visible"=w339) -> ()  [unwired: 2 in, 2 out]
          }
          frame "Relay", "Solenoid" {
            w342 = FALSE ("Visible")
            n185 = property on="Motor" class="Clust (strict)"("Visible"=w342) -> ()  [unwired: 2 in, 2 out]
            n186 = property on="Test Slider" class="Slide (strict)"("Visible"=w342) -> ()  [unwired: 2 in, 2 out]
            n187 = Search and Replace String(input string=w343, search string="/Value  **", replace string="/Direction") -> (result string=w349:string)  [unwired: 5 in, 3 out]
            n188 = property on="Test Ring" class="Ring (strict)"("Visible"=w342) -> ()  [unwired: 2 in, 2 out]
            n189 = call <vilib>:"NT Read String.vi"("Name"=w349) -> ("String"=w347:string)  [unwired: 9 in, 1 out]
            n190 = Equal?(x="Both directions", y=w347) -> (x = y?=w345:bool)
            n191 = Not(x=w345) -> (.not. x?=w346:bool)
            n192 = property on="Rev/Fwd" class="Clust (strict)"("Visible"=w345) -> ()  [unwired: 2 in, 2 out]
            n193 = property on="On/Off" class="Bool (strict)"("Visible"=w346, "Caption.Text"=w344) -> ()  [unwired: 2 in, 2 out]
          }
          frame "Compressor", "Digital Out" {
            w352 = FALSE ("Visible")
            # "Get direction and finish"
            n194 = property on="Motor" class="Clust (strict)"("Visible"=w352) -> ()  [unwired: 2 in, 2 out]
            n195 = property on="Test Slider" class="Slide (strict)"("Visible"=w352) -> ()  [unwired: 2 in, 2 out]
            n196 = property on="Test Ring" class="Ring (strict)"("Visible"=w352) -> ()  [unwired: 2 in, 2 out]
            n197 = property on="On/Off" class="Bool (strict)"("Visible"=TRUE, "Caption.Text"=w353) -> ()  [unwired: 2 in, 2 out]
            n198 = property on="Rev/Fwd" class="Clust (strict)"("Visible"=FALSE) -> ()  [unwired: 2 in, 2 out]
          }
          frame "Camera" {
            n199 = call <vilib>:"Get Last Path Segment.vi"("String in"=w360) -> ("String out"=w361:string)  [unwired: 10 in]
            n200 = property on="On/Off" class="Bool (strict)"("Visible"=FALSE) -> ()  [unwired: 2 in, 2 out]
            n201 = property on="Motor" class="Clust (strict)"("Visible"=FALSE) -> ()  [unwired: 2 in, 2 out]
            n202 = property on="Rev/Fwd" class="Clust (strict)"("Visible"=FALSE) -> ()  [unwired: 2 in, 2 out]
            n203 = case shown="\"White Balance  **\"" w361 {
              tunnel: w360 -> [w367 w376 w385 w394 w403 _ w409]
              tunnel: w359 -> [w365 w373 w382 w391 w400 _ _]
              frame "Size  **" {
                n204 = Index Array(array=w365) -> (element=w364:cluster{string[]})  [unwired: 1 in]
                n205 = call <vilib>:"NT Read String.vi"("Name"=w367) -> ("String"=w366:string)  [unwired: 9 in, 1 out]
                n206 = Unbundle(w364) -> (w362:string[])
                n207 = Match First String(2:w362, 3:w366) -> (0:w363:i32)  [unwired: 1 out]
                n208 = property on="Test Ring" class="Ring (strict)"("Value"=w363, "Strings []"=w362) -> ()  [unwired: 2 in, 2 out]
                n209 = property on="Test Ring" class="Ring (strict)"("Visible"=TRUE) -> ()  [unwired: 2 in, 2 out]
                n210 = property on="Test Slider" class="Slide (strict)"("Visible"=FALSE) -> ()  [unwired: 2 in, 2 out]
              }
              frame "White Balance  **" {
                n211 = Index Array(array=w373, index=1) -> (element=w374:cluster{string[]})
                n212 = call <vilib>:"NT Read String.vi"("Name"=w376) -> ("String"=w375:string)  [unwired: 9 in, 1 out]
                n213 = Unbundle(w374) -> (w371:string[])
                n214 = Match First String(2:w371, 3:w375) -> (0:w370:i32)  [unwired: 1 out]
                n215 = property on="Test Ring" class="Ring (strict)"("Value"=w370, "Strings []"=w371) -> ()  [unwired: 2 in, 2 out]
                n216 = property on="Test Ring" class="Ring (strict)"("Visible"=TRUE) -> ()  [unwired: 2 in, 2 out]
                n217 = property on="Test Slider" class="Slide (strict)"("Visible"=FALSE) -> ()  [unwired: 2 in, 2 out]
              }
              frame "Exposure  **" {
                n218 = Index Array(array=w382, index=2) -> (element=w383:cluster{string[]})
                n219 = call <vilib>:"NT Read String.vi"("Name"=w385) -> ("String"=w384:string)  [unwired: 9 in, 1 out]
                n220 = Unbundle(w383) -> (w379:string[])
                n221 = Match First String(2:w379, 3:w384) -> (0:w380:i32)  [unwired: 1 out]
                n222 = property on="Test Ring" class="Ring (strict)"("Value"=w380, "Strings []"=w379) -> ()  [unwired: 2 in, 2 out]
                n223 = property on="Test Ring" class="Ring (strict)"("Visible"=TRUE) -> ()  [unwired: 2 in, 2 out]
                n224 = property on="Test Slider" class="Slide (strict)"("Visible"=FALSE) -> ()  [unwired: 2 in, 2 out]
              }
              frame "Exposure Priority  **" {
                n225 = Index Array(array=w391, index=3) -> (element=w392:cluster{string[]})
                n226 = call <vilib>:"NT Read String.vi"("Name"=w394) -> ("String"=w393:string)  [unwired: 9 in, 1 out]
                n227 = Unbundle(w392) -> (w388:string[])
                n228 = Match First String(2:w388, 3:w393) -> (0:w389:i32)  [unwired: 1 out]
                n229 = property on="Test Ring" class="Ring (strict)"("Value"=w389, "Strings []"=w388) -> ()  [unwired: 2 in, 2 out]
                n230 = property on="Test Ring" class="Ring (strict)"("Visible"=TRUE) -> ()  [unwired: 2 in, 2 out]
                n231 = property on="Test Slider" class="Slide (strict)"("Visible"=FALSE) -> ()  [unwired: 2 in, 2 out]
              }
              frame "Color Enable  **" {
                n232 = Index Array(array=w400, index=4) -> (element=w401:cluster{string[]})
                n233 = call <vilib>:"NT Read String.vi"("Name"=w403) -> ("String"=w402:string)  [unwired: 9 in, 1 out]
                n234 = Unbundle(w401) -> (w397:string[])
                n235 = Match First String(2:w397, 3:w402) -> (0:w398:i32)  [unwired: 1 out]
                n236 = property on="Test Ring" class="Ring (strict)"("Value"=w398, "Strings []"=w397) -> ()  [unwired: 2 in, 2 out]
                n237 = property on="Test Ring" class="Ring (strict)"("Visible"=TRUE) -> ()  [unwired: 2 in, 2 out]
                n238 = property on="Test Slider" class="Slide (strict)"("Visible"=FALSE) -> ()  [unwired: 2 in, 2 out]
              }
              frame Default {
                n239 = property on="Test Ring" class="Ring (strict)"("Visible"=FALSE) -> ()  [unwired: 2 in, 2 out]
                n240 = property on="Test Slider" class="Slide (strict)"("Visible"=FALSE) -> ()  [unwired: 2 in, 2 out]
              }
              frame "Brightness  **", "Color Level  **", "Compression  **", "FPS  **", "Sharpness  **" {
                n241 = call <vilib>:"NT Read Number.vi"("Name"=w409) -> ("Numeric"=w408:dbl)  [unwired: 9 in, 1 out]
                n242 = local write "Test Slider"(w408) -> ()
                n243 = property on="Test Slider" class="Slide (strict)"("Visible"=TRUE, "Scale.Maximum"=100.0 ("Scale.Range:Maximum")) -> ()  [unwired: 2 in, 2 out]
                n244 = property on="Test Ring" class="Ring (strict)"("Visible"=FALSE) -> ()  [unwired: 2 in, 2 out]
              }
            }
          }
        }
        n245 = property on="Progress" class="Clust (strict)"("Visible"=FALSE) -> ()  [unwired: 2 in, 2 out]
      }
      event "Test Name": Mouse Enter {
        # "Populate the ring with the list of tests"
        n246 = event-data() -> ()  [unwired: 1 in, 1 out]
        n247 = call <vilib>:"NT Read String Array.vi"("Name"="/TestMode/TestList") -> ("String Array"=w418:string[])  [unwired: 9 in, 1 out]
        n248 = Build Array (concatenate)("Select the test to run...", w418) -> (w417:string[])
        n249 = property on="Test Name" class="Ring (strict)"("Strings []"=w417) -> ()  [unwired: 2 in, 2 out]
      }
      event "Test Name": Value Change {
        w421 = FALSE ("Visible")
        # "Tell the robot the test name to run"
        n250 = event-data() -> ("NewVal"=w425:u16)  [unwired: 1 in]
        n251 = property on="Test Name" class="Ring (strict)"() -> ("Strings []"=w426:string[])  [unwired: 2 in, 2 out]
        n252 = local write "Progress"(T5 {"Test Progress"=0, "Test Progress Text"=""} ("Progress")) -> ()
        n253 = Index Array(array=w426, index=w425) -> (element=w424:string)
        n254 = call <vilib>:"NT Write String.vi"("String"=w424, "Name"="/TestMode/TestName") -> ()  [unwired: 9 in, 1 out]
        n255 = property on="Progress" class="Clust (strict)"("Visible"=TRUE) -> ()  [unwired: 2 in, 2 out]
        n256 = property on="Motor" class="Clust (strict)"("Visible"=w421) -> ()  [unwired: 2 in, 2 out]
        n257 = property on="Test Slider" class="Slide (strict)"("Visible"=w421) -> ()  [unwired: 2 in, 2 out]
        n258 = property on="On/Off" class="Bool (strict)"("Visible"=w421) -> ()  [unwired: 2 in, 2 out]
        n259 = property on="Rev/Fwd" class="Clust (strict)"("Visible"=w421) -> ()  [unwired: 2 in, 2 out]
        n260 = property on="Test Ring" class="Ring (strict)"("Visible"=w421) -> ()  [unwired: 2 in, 2 out]
      }
      event "Select Auto": Mouse Enter {
        # "Populate the combo box with the list of autonomous options"
        n261 = event-data() -> ()  [unwired: 1 in, 1 out]
        n262 = call <vilib>:"NT Read String Array.vi"("Name"="Auto List") -> ("String Array"=w428:string[])  [unwired: 9 in, 1 out]
        n263 = property on="Select Auto" class="CmbBox"("Strings[]"=w428) -> ()  [unwired: 2 in, 2 out]
      }
      event "Select Auto": Value Change {
        # "User modified the Auto Selection. Write to NT variable so robot knows."
        n264 = event-data() -> ("NewVal"=w432:string)  [unwired: 1 in]
        n265 = call <vilib>:"NT Write String.vi"("String"=w432, "Name"="Auto Selector") -> ()  [unwired: 9 in, 1 out]
      }
      event "Command Selection": Value Change {
        # "Get the params and show in table"
        n266 = event-data() -> ("NewVal"=w439:i32)  [unwired: 1 in]
        n267 = property on="Command Selection" class="MCListbox (strict)"() -> ("ItemNames"=w437:string[][])  [unwired: 2 in, 2 out]
        n268 = call <vilib>:"WPI_DashboardUpdate Command Params.vi"("NewVal"=w439, "Commands"=w437, "Param Tbl"=w438) -> ()  [unwired: 8 in, 1 out]
      }
      event "Execute Command": Value Change {
        # "Started one, Unique ID holds\nresponse"
        n269 = event-data() -> ()  [unwired: 1 in, 1 out]
        n270 = property on="Command Selection" class="MCListbox (strict)"() -> ("ItemNames"=w451:string[][])  [unwired: 2 in, 2 out]
        n271 = Index Array(array=w451, index (row)="Command Selection", index (col)=0) -> (element=w449:string)
        n272 = call <vilib>:"Invoke Commands.vi"("Command Params"="Command Params", "Function Name"=w449) -> ("Params"=w445:u8, "Started"=w444:bool)  [unwired: 7 in, 1 out]
        n273 = Array Subset(array="Command Params", length (row)=w445) -> (w446:string[][])  [unwired: 3 in]
        n274 = Select(t="Executing" ("Cmd Status"), s=w444, f="" ("Cmd Status")) -> (s? t:f=→"Cmd Status":string)
      }
      event "Command Selection": Double Click {
        n275 = event-data() -> ("Row"=w461:i32)  [unwired: 1 in]
        n276 = property on="Command Selection" class="MCListbox (strict)"() -> ("ItemNames"=w464:string[][])  [unwired: 2 in, 2 out]
        n277 = local read "Command Params"() -> (w459:string[][])
        n278 = Index Array(array=w464, index (row)=w461, index (col)=0) -> (element=w462:string)
        n279 = call <vilib>:"Invoke Commands.vi"("Command Params"=w459, "Function Name"=w462) -> ("Params"=w458:u8, "Started"=w453:bool)  [unwired: 7 in, 1 out]
        n280 = Array Subset(array=w459, length (row)=w458) -> (w457:string[][])  [unwired: 3 in]
        n281 = Select(t="Executing" ("Cmd Status"), s=w453, f="" ("Cmd Status")) -> (s? t:f=w454:string)
        n282 = local write "Cmd Status"(w454) -> ()
      }
      event "CheckList": Double Click {
        # "Shift clears all"
        # "Update symbols on the listbox"
        n283 = event-data() -> ("PlatMods.Shift"=w467:bool, "Row"=w469:i32)  [unwired: 1 in]
        n284 = case shown="True" w467 {
          tunnel: w469 -> [w473 _]
          tunnel: 1 -> [w472 _]
          frame False {
            n285 = property on="CheckList" class="LstBox (strict)"() -> ("Item Symbols"=w471:i32[])  [unwired: 2 in, 2 out]
            n286 = Replace Array Subset(array=w471, new element=w472, index=w473) -> (w470:i32[])
            n287 = property on="CheckList" class="LstBox (strict)"("Item Symbols"=w470) -> ()  [unwired: 2 in, 2 out]
          }
          frame True {
            w474 = 0 ("Top Row")
            n288 = property on="CheckList" class="LstBox (strict)"() -> ("Number of Rows"=w476:u32)  [unwired: 2 in, 2 out]
            n289 = Initialize Array(0, w476) -> (w475:i32[])
            n290 = property on="CheckList" class="LstBox (strict)"("Top Row"=w474, "Value"=w474, "Item Symbols"=w475) -> ()  [unwired: 2 in, 2 out]
          }
        }
      }
      event "CheckList": Key Down {
        # "Update symbols on the listbox\nLeft and right keys check and uncheck"
        n291 = event-data() -> ("VKey"=w481:T27)  [unwired: 1 in]
        n292 = case shown="\"Left\", \"Right\"" w481 {
          selector: w481 -> [w486 _]
          tunnel: eventvkey."Left" ("VKey") -> [w484 _]
          frame "Left", "Right" {
            n293 = Equal?(x=w484, y=w486) -> (x = y?=w485:bool)
            n294 = Select(t=0, s=w485, f=1) -> (s? t:f=w487:i32)
            n295 = property on="CheckList" class="LstBox (strict)"() -> ("Item Symbols"=w490:i32[])  [unwired: 2 in, 2 out]
            n296 = Replace Array Subset(array=w490, new element=w487, index="CheckList") -> (w489:i32[])
            n297 = property on="CheckList" class="LstBox (strict)"("Item Symbols"=w489) -> ()  [unwired: 2 in, 2 out]
          }
          frame Default {
          }
        }
      }
      event "DB Camera Config": Value Change {
        # "Show or hide the cluster of controls, store in ini file"
        n298 = event-data() -> ("NewVal"=w495:bool)  [unwired: 1 in]
        n299 = case shown="False" w495 {
          tunnel: w494 -> [w504 _]
          tunnel: [w497 w515] -> w493
          tunnel: w492 -> [w496 w515]
          frame False {
            w511 = "Camera"
            w514 = FALSE ("Visible")
            n300 = local read "Camera Settings"() -> (w503:T2)
            n301 = Index Array(array=w504) -> (element=w507:cluster{string[]})  [unwired: 1 in]
            n302 = Unbundle(w503) -> ("Frame Rate"=w502:i32, "Compression"=w501:i32, "Size"=w505:u16)
            n303 = Unbundle(w507) -> (w506:string[])
            n304 = Index Array(array=w506, index=w505) -> (element=w500:string)
            n305 = call-poly <vilib>:"Write Key.vi"("section"=w511, "value"=w500, "key"="Size", "refnum"=w496) -> ("refnum out"=w513:T21)  [unwired: 2 in, 5 out]
            n306 = call-poly <vilib>:"Write Key.vi"("section"=w511, "value"=w502, "key"="FrameRate", "refnum"=w513) -> ("refnum out"=w512:T21)  [unwired: 1 in, 6 out]
            n307 = property on="Camera Settings" class="Clust (strict)"("Visible"=w514) -> ()  [unwired: 2 in, 2 out]
            n308 = local write "DB Camera Config"(w514) -> ()
            n309 = call-poly <vilib>:"Write Key.vi"("section"=w511, "value"=w501, "key"="Compression", "refnum"=w512) -> ("refnum out"=w498:T21)  [unwired: 1 in, 6 out]
            n310 = call <vilib>:"Close Config Data.vi"("refnum"=w498) -> ("file path"=w499:path)  [unwired: 2 in, 8 out]
            n311 = call <vilib>:"Open Config Data.vi"("configuration file path"=w499) -> ("refnum"=w497:T21)  [unwired: 8 in, 2 out]
          }
          frame True {
            n312 = property on="Camera Settings" class="Clust (strict)"("Visible"=TRUE) -> ()  [unwired: 2 in, 2 out]
          }
        }
      }
      event "Camera Settings": Value Change {
        # "Update summary string when any elements of DB camera change"
        n313 = event-data() -> ("NewVal"=w529:T2)  [unwired: 1 in]
        n314 = Index Array(array=w525) -> (element=w524:cluster{string[]})  [unwired: 1 in]
        n315 = Unbundle(w529) -> ("Frame Rate"=w520:i32, "Compression"=w519:i32, "Size"=w522:u16)
        n316 = Unbundle(w524) -> (w523:string[])
        n317 = Index Array(array=w523, index=w522) -> (element=w521:string)
        n318 = Format Into String(format string="%s   %dfps   %d%%", w521, w520, w519) -> (resulting string=w526:string)  [unwired: 2 in, 1 out]
        n319 = Build Array(w526) -> (w527:string[])
        n320 = property on="DB Camera Config" class="Bool (strict)"("Strings [4]"=w527) -> ()  [unwired: 2 in, 2 out]
      }
      event "Motor.Enable": Value Change {
        # "When the test mode otor enable helper is set, update that\ntree row item's value"
        n321 = event-data() -> ("NewVal"=w536:bool)  [unwired: 1 in]
        n322 = Unbundle("Motor") -> ("Value"=w535:dbl)  [unwired: 1 out]
        n323 = Select(t=w535, s=w536, f=0.0) -> (s? t:f=w533:dbl)
        n324 = call <vilib>:"NT Write Number.vi"("Numeric"=w533, "Name"=w532) -> ()  [unwired: 9 in, 1 out]
      }
      event "Test Slider": Value Change {
        # "When the test mode slider helper is set, update that\ntree row item's value"
        n325 = event-data() -> ("NewVal"=w540:dbl)  [unwired: 1 in]
        n326 = call <vilib>:"NT Write Number.vi"("Numeric"=w540, "Name"=w541) -> ()  [unwired: 9 in, 1 out]
      }
      event "On/Off": Value Change {
        # "When the test mode on/off helper value is set, update that\ntree row item's value"
        n327 = event-data() -> ("NewVal"=w546:bool)  [unwired: 1 in]
        n328 = Boolean To (0,1)(Boolean=w546) -> (0, 1=w545:i16)
        n329 = call <vilib>:"NT Write Number.vi"("Numeric"=w545, "Name"=w544) -> ()  [unwired: 9 in, 1 out]
      }
      event "Rev/Fwd": Value Change {
        # "When the test mode helper value for relays is set, update that\ntree row item's value"
        n330 = event-data() -> ("NewVal.Forward"=w555:bool, "NewVal.Reverse"=w554:bool)  [unwired: 1 in]
        n331 = Boolean To (0,1)(Boolean=w555) -> (0, 1=w551:i16)
        n332 = Boolean To (0,1)(Boolean=w554) -> (0, 1=w553:i16)
        n333 = Negate(x=w553) -> (-x=w552:i16)
        n334 = Add(x=w551, y=w552) -> (x+y=w550:i16)
        n335 = call <vilib>:"NT Write Number.vi"("Numeric"=w550, "Name"=w549) -> ()  [unwired: 9 in, 1 out]
      }
      event "Test Ring": Value Change {
        # "When a test mode helper value is selected from the ring,\nset the tree item's variable to the string value"
        n336 = event-data() -> ("NewVal"=w560:u16)  [unwired: 1 in]
        n337 = property on="Test Ring" class="Ring (strict)"() -> ("Strings []"=w561:string[])  [unwired: 2 in, 2 out]
        n338 = Index Array(array=w561, index=w560) -> (element=w559:string)
        n339 = call <vilib>:"NT Write String.vi"("String"=w559, "Name"=w558) -> ()  [unwired: 9 in, 1 out]
      }
      event "Rec Mode": Value Change {
        # "Update globals for recording mode and path to read log from.\nClear when logging and let NetworkTables set path for vision to\nuse."
        n340 = event-data() -> ("NewVal"=w573:enum32{"Stop", "Record", "Playback"})  [unwired: 1 in]
        n341 = global write "WPI_DashboardLogging Global.vi" "Logging Filename"(path "") -> ()
        n342 = global write "WPI_DashboardLogging Global.vi" "Recording"(w573) -> ()
        n343 = case shown="\"Playback\"" w573 {
          tunnel: w572 -> [_ w575 w584]
          tunnel: [_ _ w583] -> w569
          tunnel: [_ _ w582] -> _
          tunnel: w567 -> [_ _ w580]
          tunnel: cluster{i32, i32} {-250, 170} -> [_ _ w579]
          tunnel: [_ _ T28 {"Image Size"=TRUE, "Image Type"=TRUE, "Pixel Value"=TRUE, "ROI Information"=TRUE, "Zoom Factor"=FALSE} ("Image Information Shown:All Elements")] -> w565
          tunnel: [_ _ TRUE ("Zoom Factor")] -> w564
          tunnel: w563 -> [_ _ w576]
          frame Default {
          }
          frame "Stop", "Record" {
            # "Place Window too"
            n344 = invoke class="VI" method="FP.Close"(reference=w575) -> (reference out=w574:refnum<vi>)  [unwired: 2 in, 2 out]
            n345 = invoke class="VI" method="Abort VI"(reference=w574) -> ()  [unwired: 2 in, 3 out]
          }
          frame "Playback" {
            n346 = call "Open Playback Panel.vi"("Offset"=w579, "DB VI Ref"=w580, "Playback in"=w584) -> ("Playback out"=w581:refnum<vi>)  [unwired: 8 in]
            n347 = register-events(w581, w576) -> (reference out=w583:refnum<event-registration>, error out=w582:errorcluster)  [unwired: 2 in]
          }
        }
        n348 = property on="Camera Image" class="ImageControl"("Image Information Shown"=w565, "Image Information Visible"=w564) -> ()  [unwired: 2 in, 2 out]
        n349 = call <vilib>:"WPI_DashboardNT Log FieldName Cache.vi"("Operation"=enum16{"Lookup/Add", "Index", "Clear"}."Clear") -> ()  [unwired: 8 in, 3 out]
      }
      event Panel Close {
        w586 = enum32{"Stop", "Record", "Playback"}."Stop" ("Rec Mode")
        # "Playback window has been closed, abort"
        n350 = event-data() -> ()  [unwired: 1 in, 4 out]
        n351 = local write "Rec Mode"(w586) -> ()
        n352 = global write "WPI_DashboardLogging Global.vi" "Recording"(w586) -> ()
      }
      event Panel Close {
        # "Abort playback window and ourself"
        n353 = event-data() -> ()  [unwired: 1 in, 4 out]
        n354 = invoke class="VI" method="FP.Close"(reference=w592) -> (reference out=w591:refnum<vi>)  [unwired: 2 in, 2 out]
        n355 = invoke class="VI" method="Abort VI"(reference=w591) -> (error out=w590:errorcluster)  [unwired: 2 in, 2 out]
        n356 = invoke class="VI" method="Abort VI"(error in=w590) -> ()  [unwired: 2 in, 3 out]
      }
      event User Event {
        n357 = event-data() -> ("IDs"=w600:cluster{"RPC field ID":u16, "Unique ID":u16}, "String"=w599:string)  [unwired: 1 in]
        n358 = Bundle("IDs"=w600, "String"=w599) -> (w598:T12)  [unwired: 1 in]
        n359 = call <vilib>:"Retrieve RPC Response.vi"("RPC Response"=w598) -> ("Output"=w595:string[][])  [unwired: 10 in]
        n360 = Build Array (concatenate)(w593, w595) -> (w594:string[][])
        n361 = local write "Command Params"(w594) -> ()
        n362 = local write "Cmd Status"("" ("Cmd Status")) -> ()
      }
      event "Vision": Value Change {
        # "Enable/Disable Compression slider.\nHW USB is hard-coded into the camera"
        n363 = event-data() -> ("NewVal"=w607:u16)  [unwired: 1 in]
        n364 = Equal?(x=w607, y=u32 2 ("milliseconds to wait")) -> (x = y?=w605:bool)
        n365 = Select(t=T29."Disabled and Grayed Out" ("Disabled"), s=w605, f=T29."Enabled" ("Disabled")) -> (s? t:f=w602:T29)
        n366 = property on="Compression" class="Slide (strict)"("DisabledEnum"=w602) -> ()  [unwired: 2 in, 2 out]
      }
      event "Tree": Double Click {
        n367 = event-data() -> ("PlatMods"=w612:T32, "Tag"=w611:string)  [unwired: 1 in]
        n368 = Unbundle(w612) -> ("Shift"=w610:bool)  [unwired: 4 out]
        n369 = Not(x=w610) -> (.not. x?=w609:bool)
        n370 = call <vilib>:"NT Update Persistence.vi"("Persistence"=w609, "Name"=w611) -> ()  [unwired: 9 in, 1 out]
      }
    }
  }
  n371 = while {
    tunnel: w66 -> [w616]
    i -> [w619]
    stop <- FALSE stop-if-true
    n372 = Wait (ms)(milliseconds to wait=u32 100) -> ()  [unwired: 1 out]
    n373 = case shown="\"Playback\"" "Rec Mode" {
      tunnel: w619 -> [_ _ w634]
      tunnel: [u32 2829099 ("Base Color") u32 11141120 ("Target Color") w623] -> w615
      frame "Stop", Default {
        # "Reset the color, extra updates don't cost much"
      }
      frame "Record" {
      }
      frame "Playback" {
        # "Playback"
        n374 = Quotient & Remainder(x=w634, y=u32 50 ("milliseconds to wait")) -> (x-y*floor(x/y)=w630:u32)  [unwired: 1 out]
        n375 = Divide(x=w630, y=u32 50 ("milliseconds to wait")) -> (x/y=w627:dbl)
        n376 = Multiply(x=6.283185307179586, y=w627) -> (x*y=w632:dbl)
        n377 = Sine(x=w632) -> (sin(x)=w631:dbl)
        n378 = Absolute Value(x=w631) -> (abs(x)=w624:dbl)
        n379 = call "Interpolate RGB Color.vi"("Proportion"=w624, "Target Color"=u32 30976, "Base Color"=u32 2829099) -> ("Result Color"=w623:u32)  [unwired: 8 in]
      }
    }
    n380 = property class="Pane"(reference=w616, "PaneColor"=w615) -> ()  [unwired: 1 in, 2 out]
  }
  n381 = property on="On/Off" class="Bool (strict)"("Visible"=w34) -> ()  [unwired: 2 in, 2 out]
  n382 = property on="Motor" class="Clust (strict)"("Visible"=w34) -> ()  [unwired: 2 in, 2 out]
  n383 = property on="Progress" class="Clust (strict)"("Visible"=w34) -> ()  [unwired: 2 in, 2 out]
  n384 = property on="Test Ring" class="Ring (strict)"("Visible"=w34) -> ()  [unwired: 2 in, 2 out]
  n385 = property on="Rev/Fwd" class="Clust (strict)"("Visible"=w34) -> ()  [unwired: 2 in, 2 out]
  n386 = property on="Camera Settings" class="Clust (strict)"("Visible"=w34) -> ()  [unwired: 2 in, 2 out]
  n387 = local write "DB Camera Config"(w34) -> ()
  n388 = local write "Command Params"(string[][] [] ("Command Params")) -> ()
  n389 = global write "WPI_DashboardLogging Global.vi" "Recording"(w60) -> ()
  n390 = local write "Rec Mode"(w60) -> ()
  n391 = while {
    tunnel: u16 1741 ("timeout ms (25000)") -> [w636]
    stop <- FALSE stop-if-true
    n392 = TCP Create Listener(10:w636) -> (0:w635:errorcluster, 3:w637:refnum<k5>)  [unwired: 4 in, 1 out]
    n393 = case shown="No Error" w635 {
      selector: w635 -> [w639 _]
      tunnel: w637 -> [w640 _]
      frame No Error {
        n394 = while {
          tunnel: w640 -> [w643]
          tunnel: w639 -> [w642]
          stop <- FALSE stop-if-true
          n395 = TCP Wait On Listener(8:w642, 11:w643) -> (0:w644:errorcluster, 4:w645:refnum<k5>)  [unwired: 2 in, 3 out]
          n396 = local write "TCP"(w645) -> ()
          n397 = case shown="No Error" w644 {
            frame No Error {
            }
            frame Error {
              n398 = Wait (ms)(milliseconds to wait=u32 1000) -> ()  [unwired: 1 out]
            }
          }
        }
      }
      frame Error {
        n399 = Wait (ms)(milliseconds to wait=u32 1000) -> ()  [unwired: 1 out]
      }
    }
  }
  n400 = local write "Command Selection"(u16 0 ("milliseconds to wait")) -> ()
